vi "Semi_Random.vi"() -> ()   [LabVIEW 2017]
uses:
  <vilib>/Analysis/baseanly.llb/Mean (DBL).vi
  <vilib>/Analysis/NI_AALBase.lvlib
panel:
  in  "stop":bool
  out "Waveform Chart":cluster{"number: 0 to 1":dbl, "mean":dbl}(graph)
  out "Array 2":u32[](array[colorbox])
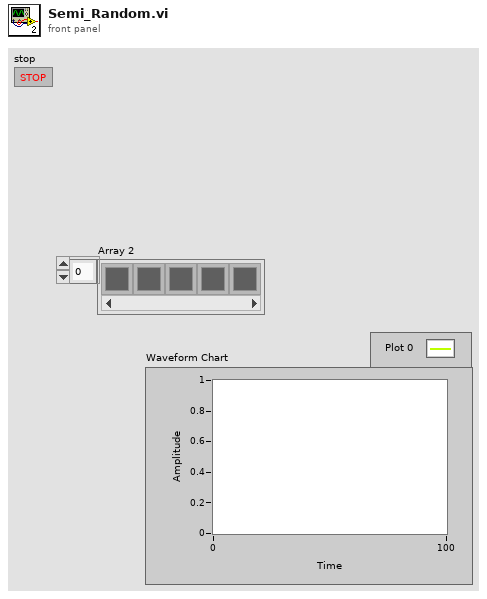
[diagram p1: front panel]
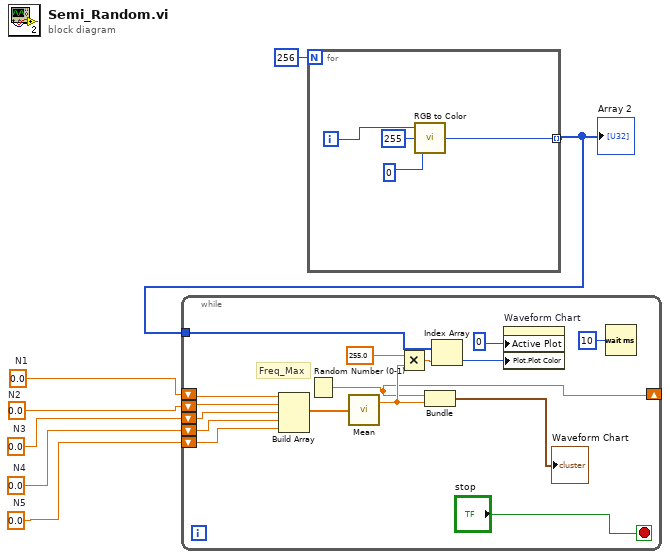
[diagram p0: block diagram]
diagram:
  w2 = 0.0  # N5
  w3 = 0.0  # N4
  w4 = 0.0  # N3
  w5 = 0.0  # N2
  w6 = 0.0  # N1
  n1 = for {
    N: 256 -> [_]
    tunnel: [w10] -> w1 mode=indexing
    i -> [w11]
    n2 = call <vilib>:"RGB to Color.vi"("B"=u8 0, "G"=u8 255, "R"=w11) -> ("Color"=w10:u32)
  }
  "Array 2" <- w1
  n3 = while {
    shift-right: [w12] -> _
    shift-left: w6 -> [w26]
    shift-left: w5 -> [w25]
    shift-left: w4 -> [w24]
    shift-left: w3 -> [w23]
    shift-left: w2 -> [w22]
    tunnel: w1 -> [w18]
    stop <- "stop" stop-if-true
    # "Freq_Max"
    n4 = Build Array(w26, w25, w24, w23, w22) -> (w21:dbl[])
    n5 = Random Number (0-1)() -> (number: 0 to 1=w12:dbl)
    n6 = call-poly <vilib>:"Mean.vi"("X"=w21) -> ("mean"=w13:dbl)  [unwired: 1 out]
    n7 = Multiply(x=255.0, y=w13) -> (x*y=w19:dbl)
    n8 = Bundle("number: 0 to 1"=w12, "mean"=w13) -> (→"Waveform Chart":cluster{"number: 0 to 1":dbl, "mean":dbl})  [unwired: 1 in]
    n9 = Index Array(array=w18, index=w19) -> (element=w16:u32)
    n10 = property on="Waveform Chart" class="WFChart (strict)"("Active Plot"=0, "Plot.Plot Color"=w16) -> ()  [unwired: 2 in, 2 out]
    n11 = Wait (ms)(milliseconds to wait=u32 10) -> ()  [unwired: 1 out]
  }
